vi "Arm Transfer F to R.vi"() -> ()   [LabVIEW 2015]
uses:
  Typedef/IntakeControllerActions.ctl
  Typedef/IntakeControllerMsg.ctl
  ArmController/ArmController.lvlib
panel:
  in  "milliseconds to wait 2":u32=500
  in  "milliseconds to wait":u32=250
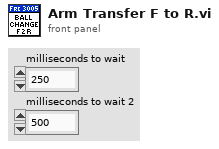
[diagram p1: front panel]
types:
  T1 = typedef "IntakeControllerMsg.ctl" = cluster{"Cmd":T2, "Data":variant}
  T2 = typedef "IntakeControllerActions.ctl" = enum16{"Wait on Intake Rear", "Wait on Angle Rear", "Go To Angle Rear", "Wait on Intake Front", "Wait on Angle Front", "Set Roller Front", "Set Roller Rear", "Go To Angle Front", "Wait ms"}
  T3 = cluster{"Down":dbl, "Pickup":dbl, "Shoot":dbl, "Turtle":dbl, "Intake Block":dbl, "Intake Transfer":dbl}
  T4 = cluster{"Down":dbl, "Pickup":dbl, "Shoot":dbl, "Turtle":dbl}
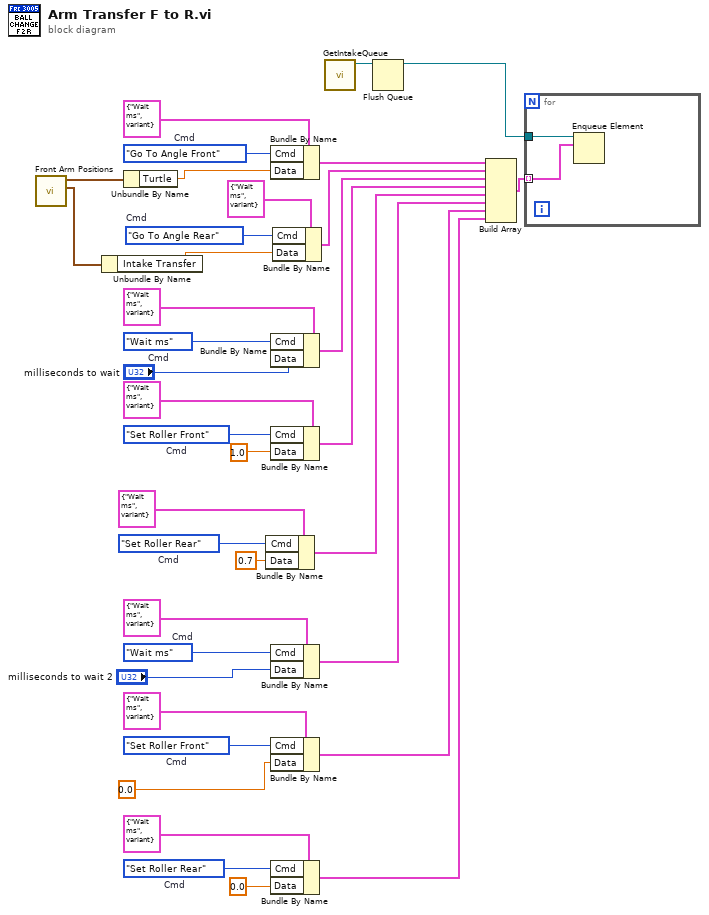
[diagram p0: block diagram]
diagram:
  w4 = IntakeControllerActions."Set Roller Rear"  # Cmd
  w11 = IntakeControllerActions."Go To Angle Rear"  # Cmd
  w37 = IntakeControllerActions."Set Roller Rear"  # Cmd
  w29 = IntakeControllerActions."Set Roller Front"  # Cmd
  w33 = IntakeControllerActions."Wait ms"  # Cmd
  w26 = IntakeControllerActions."Set Roller Front"  # Cmd
  w21 = IntakeControllerActions."Wait ms"  # Cmd
  w18 = IntakeControllerActions."Go To Angle Front"  # Cmd
  n1 = call "Front Arm Positions.vi"() -> ("Rear Arm"=w8:T3, "Front Arm"=w13:T4)  [unwired: 10 in]
  n2 = Unbundle By Name(w8) -> ("Intake Transfer"=w7:dbl)
  n3 = Unbundle By Name(w13) -> ("Turtle"=w14:dbl)
  n4 = Bundle By Name(cluster=T1 {"Cmd"=enum."Wait ms", "Data"=variant(i32 50)} ("output cluster"), "Cmd"=w4, "Data"=0.7) -> (w2:T1)
  n5 = Bundle By Name(cluster=T1 {"Cmd"=enum."Wait ms", "Data"=variant(i32 50)} ("output cluster"), "Cmd"=w18, "Data"=w14) -> (w20:T1)
  n6 = Bundle By Name(cluster=T1 {"Cmd"=enum."Wait ms", "Data"=variant(i32 50)} ("output cluster"), "Cmd"=w21, "Data"="milliseconds to wait") -> (w24:T1)
  n7 = Bundle By Name(cluster=T1 {"Cmd"=enum."Wait ms", "Data"=variant(i32 50)} ("output cluster"), "Cmd"=w26, "Data"=1.0) -> (w27:T1)
  n8 = Bundle By Name(cluster=T1 {"Cmd"=enum."Wait ms", "Data"=variant(i32 50)} ("output cluster"), "Cmd"=w33, "Data"="milliseconds to wait 2") -> (w1:T1)
  n9 = Bundle By Name(cluster=T1 {"Cmd"=enum."Wait ms", "Data"=variant(i32 50)} ("output cluster"), "Cmd"=w29, "Data"=0.0 ("Diffs")) -> (w35:T1)
  n10 = Bundle By Name(cluster=T1 {"Cmd"=enum."Wait ms", "Data"=variant(i32 50)} ("output cluster"), "Cmd"=w37, "Data"=0.0 ("Diffs")) -> (w16:T1)
  n11 = Bundle By Name(cluster=T1 {"Cmd"=enum."Wait ms", "Data"=variant(i32 50)} ("output cluster"), "Cmd"=w11, "Data"=w7) -> (w9:T1)
  n12 = call "GetIntakeQueue.vi"() -> ("queue out"=w17:refnum<queue>)  [unwired: 11 in]
  n13 = Flush Queue(queue=w17) -> (queue out=w15:refnum<queue>)  [unwired: 1 in, 2 out]
  n14 = Build Array(w20, w9, w24, w27, w2, w1, w35, w16) -> (w28:T1[])
  n15 = for {
    tunnel: w15 -> [w39]
    tunnel: w28 -> [w38] mode=indexing
    n16 = Enqueue Element(queue=w39, element=w38) -> ()  [unwired: 2 in, 3 out]
  }
